vi "byte40-41 (SubVI).vi"(11 "unsigned byte array":u8[](array[numeric])) -> (0 "Numeric":dbl, 1 "Boolean":bool, 2 "Boolean 2":bool, 3 "Boolean 3":bool)   [LabVIEW 2016]
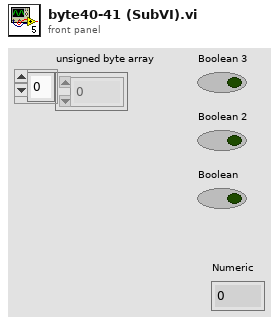
[diagram p1: front panel]
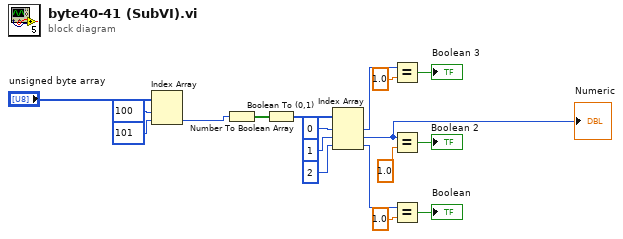
[diagram p0: block diagram]
diagram:
  n1 = Index Array(array="unsigned byte array", index #1=100 ("index"), index #2=101 ("index")) -> (element #2=w2:u8)  [unwired: 1 out]
  n2 = Number To Boolean Array(number=w2) -> (Boolean array=w6:bool[])
  n3 = Boolean To (0,1)(Boolean=w6) -> (0, 1=w7:i16[])
  n4 = Index Array(array=w7, index #1=0 ("index"), index #2=1 ("index"), index #3=2 ("index")) -> (element #1=w12:i16, element #2=w1:i16, element #3=w17:i16)
  "Numeric" <- w1
  n5 = Equal?(x=w12, y=1.0) -> (x = y?=→"Boolean 3":bool)
  n6 = Equal?(x=w1, y=1.0) -> (x = y?=→"Boolean 2":bool)
  n7 = Equal?(x=w17, y=1.0) -> (x = y?=→"Boolean":bool)
